vi "ULx Start Task.vi"(0 "task in":refnum<k24>, 11 "error in":errorcluster) -> (4 "task out":refnum<k24>, 15 "error out":errorcluster)   [LabVIEW 2020]
doc: "Transitions the task to the running state to begin the measurement or generation. Using this VI is required for some applications and is optional for others."
uses:
  C:/Users/William/Documents/LV 2020 builds/LeaktestDAQ/Source-v33/ULx_LV.dll
  ULx_LV.dll
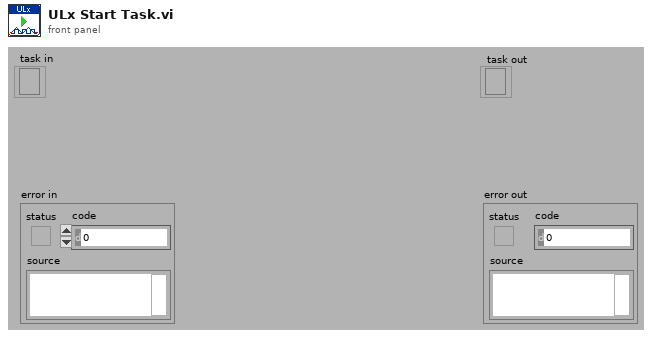
[diagram p1: front panel]
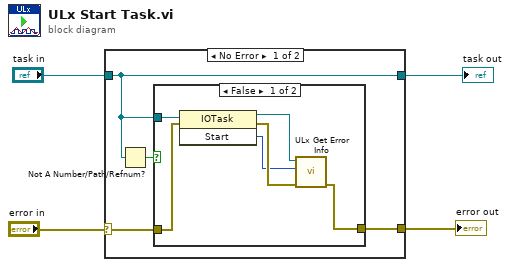
[diagram p0: block diagram]
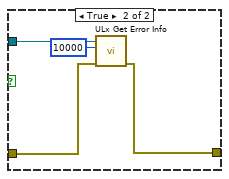
[diagram p2: hidden frame]
diagram:
  n1 = case shown="No Error" "error in" {
    selector: "error in" -> [w7 w20]
    tunnel: "task in" -> [w5 w19]
    tunnel: [w8 w20] -> w2
    tunnel: [w5 w19] -> w1
    frame No Error {
      n2 = Not A Number/Path/Refnum?(number/path/refnum=w5) -> (NaN/Path/Refnum?=w6:bool)
      n3 = case shown="False" w6 {
        tunnel: w5 -> [w14 w17]
        tunnel: [w12 w15] -> w8
        tunnel: w7 -> [w10 w16]
        frame False {
          n4 = invoke class="IOTask" method="Start"(reference=w14, error in=w10) -> (reference out=w13:refnum<k24>, error out=w11:errorcluster, "Start"=w9:i32)  [unwired: 1 in]
          n5 = call "ULx Get Error Info.vi"("error in"=w11, "ErrorCode"=w9, "task in"=w13) -> ("error out"=w12:errorcluster)  [unwired: 8 in]
        }
        frame True {
          n6 = call "ULx Get Error Info.vi"("error in"=w16, "ErrorCode"=10000, "task in"=w17) -> ("error out"=w15:errorcluster)  [unwired: 8 in]
        }
      }
    }
    frame Error {
    }
  }
  "error out" <- w2
  "task out" <- w1
